vi "WriteLog.vi"(8 "Online Eye Model":T2, 10 "Current System State":T1(ring), 11 "File In":refnum<file>) -> (3 "File Out":refnum<file>)   [LabVIEW 2016]
uses:
  Subsystems/Global Variables.vi
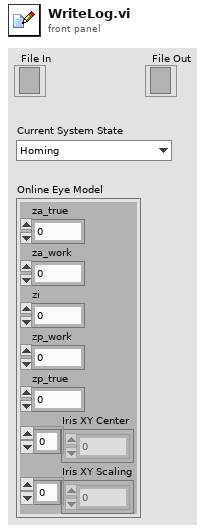
[diagram p1: front panel]
types:
  T1 = enum16{"Homing", "M/S Initialization", "M/S Operation", "Aiming", "Engaging", "Trajectory Loading", "Tracking Initialization", "Tracking", "Rerouting", "Regulation"}
  T2 = cluster{"za_true":dbl, "za_work":dbl, "zi":dbl, "zp_work":dbl, "zp_true":dbl, "Iris XY Center":dbl[], "Iris XY Scaling":dbl[]}
  T3 = cluster{"Accurus button":bool[], "Accurus engaged?":bool, "Vacuum Force":i32, "Accurus Ch. A Vout":dbl, "Accurus Ch. B Vout":dbl, "Irrigation engaged?":bool}
  T4 = cluster{"Iris XY Center[0]":dbl, "Iris XY Center[1]":dbl, "Iris XY Center[2]":dbl, "Iris XY Center[3]":dbl, "Iris XY Center[4]":dbl, "Iris XY Center[5]":dbl, "Iris XY Center[6]":dbl, "Iris XY Center[7]":dbl, "Iris XY Center[8]":dbl}
  T5 = cluster{"Iris XY Scaling[0]":dbl, "Iris XY Scaling[1]":dbl, "Iris XY Scaling[2]":dbl, "Iris XY Scaling[3]":dbl, "Iris XY Scaling[4]":dbl, "Iris XY Scaling[5]":dbl, "Iris XY Scaling[6]":dbl, "Iris XY Scaling[7]":dbl, "Iris XY Scaling[8]":dbl}
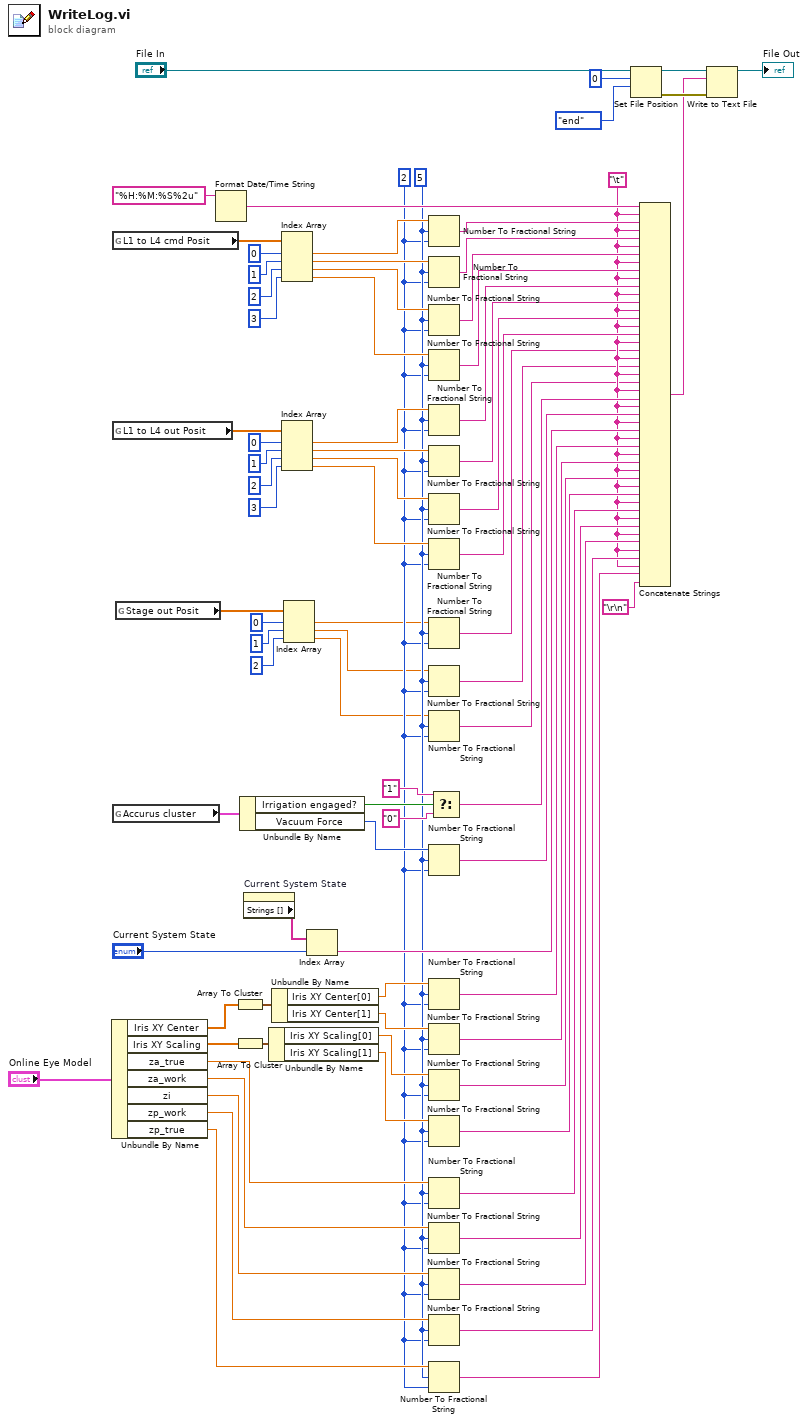
[diagram p0: block diagram]
diagram:
  w7 = 2
  w8 = 5
  w13 = "\t"
  n1 = Unbundle By Name("Online Eye Model") -> ("Iris XY Center"=w37:dbl[], "Iris XY Scaling"=w34:dbl[], "za_true"=w29:dbl, "za_work"=w28:dbl, "zi"=w27:dbl, "zp_work"=w26:dbl, "zp_true"=w25:dbl)
  n2 = global read "Global Variables.vi" "L1 to L4 cmd Posit"() -> (w69:dbl[])
  n3 = global read "Global Variables.vi" "L1 to L4 out Posit"() -> (w52:dbl[])
  n4 = global read "Global Variables.vi" "Accurus cluster"() -> (w47:T3)
  n5 = global read "Global Variables.vi" "Stage out Posit"() -> (w12:dbl[])
  n6 = Format Date/Time String(time format string (%c)="%H:%M:%S%2u") -> (date/time string=w74:string)  [unwired: 2 in]
  n7 = Array To Cluster(array=w37) -> (cluster=w36:T4)
  n8 = Array To Cluster(array=w34) -> (cluster=w35:T5)
  n9 = Unbundle By Name(w47) -> ("Irrigation engaged?"=w45:bool, "Vacuum Force"=w46:i32)
  n10 = property on="Current System State" class="Enum (strict)"() -> ("Strings []"=w41:string[])  [unwired: 2 in, 2 out]
  n11 = Unbundle By Name(w35) -> ("Iris XY Scaling[0]"=w31:dbl, "Iris XY Scaling[1]"=w30:dbl)
  n12 = Unbundle By Name(w36) -> ("Iris XY Center[0]"=w33:dbl, "Iris XY Center[1]"=w32:dbl)
  n13 = Index Array(array=w69, index #1=0 ("index"), index #2=1 ("index"), index #3=2 ("index"), index #4=3 ("index")) -> (element #1=w68:dbl, element #2=w61:dbl, element #3=w67:dbl, element #4=w66:dbl)
  n14 = Index Array(array=w52, index #1=0 ("index"), index #2=1 ("index"), index #3=2 ("index"), index #4=3 ("index")) -> (element #1=w54:dbl, element #2=w53:dbl, element #3=w59:dbl, element #4=w60:dbl)
  n15 = Index Array(array=w12, index #1=0 ("index"), index #2=1 ("index"), index #3=2 ("index")) -> (element #1=w6:dbl, element #2=w5:dbl, element #3=w4:dbl)
  n16 = Index Array(array=w41, index="Current System State") -> (element=w39:string)
  n17 = Number To Fractional String(number=w68, width (-)=w8, precision (6)=w7) -> (F-format string=w65:string)  [unwired: 1 in]
  n18 = Number To Fractional String(number=w61, width (-)=w8, precision (6)=w7) -> (F-format string=w64:string)  [unwired: 1 in]
  n19 = Number To Fractional String(number=w67, width (-)=w8, precision (6)=w7) -> (F-format string=w63:string)  [unwired: 1 in]
  n20 = Number To Fractional String(number=w66, width (-)=w8, precision (6)=w7) -> (F-format string=w62:string)  [unwired: 1 in]
  n21 = Number To Fractional String(number=w54, width (-)=w8, precision (6)=w7) -> (F-format string=w51:string)  [unwired: 1 in]
  n22 = Number To Fractional String(number=w53, width (-)=w8, precision (6)=w7) -> (F-format string=w50:string)  [unwired: 1 in]
  n23 = Number To Fractional String(number=w59, width (-)=w8, precision (6)=w7) -> (F-format string=w49:string)  [unwired: 1 in]
  n24 = Number To Fractional String(number=w60, width (-)=w8, precision (6)=w7) -> (F-format string=w48:string)  [unwired: 1 in]
  n25 = Number To Fractional String(number=w6, width (-)=w8, precision (6)=w7) -> (F-format string=w3:string)  [unwired: 1 in]
  n26 = Number To Fractional String(number=w5, width (-)=w8, precision (6)=w7) -> (F-format string=w2:string)  [unwired: 1 in]
  n27 = Number To Fractional String(number=w4, width (-)=w8, precision (6)=w7) -> (F-format string=w1:string)  [unwired: 1 in]
  n28 = Number To Fractional String(number=w46, width (-)=w8, precision (6)=w7) -> (F-format string=w42:string)  [unwired: 1 in]
  n29 = Number To Fractional String(number=w33, width (-)=w8, precision (6)=w7) -> (F-format string=w24:string)  [unwired: 1 in]
  n30 = Number To Fractional String(number=w32, width (-)=w8, precision (6)=w7) -> (F-format string=w23:string)  [unwired: 1 in]
  n31 = Number To Fractional String(number=w31, width (-)=w8, precision (6)=w7) -> (F-format string=w22:string)  [unwired: 1 in]
  n32 = Number To Fractional String(number=w30, width (-)=w8, precision (6)=w7) -> (F-format string=w21:string)  [unwired: 1 in]
  n33 = Number To Fractional String(number=w29, width (-)=w8, precision (6)=w7) -> (F-format string=w20:string)  [unwired: 1 in]
  n34 = Number To Fractional String(number=w28, width (-)=w8, precision (6)=w7) -> (F-format string=w19:string)  [unwired: 1 in]
  n35 = Number To Fractional String(number=w27, width (-)=w8, precision (6)=w7) -> (F-format string=w18:string)  [unwired: 1 in]
  n36 = Number To Fractional String(number=w26, width (-)=w8, precision (6)=w7) -> (F-format string=w17:string)  [unwired: 1 in]
  n37 = Number To Fractional String(number=w25, width (-)=w8, precision (6)=w7) -> (F-format string=w16:string)  [unwired: 1 in]
  n38 = Select(t="1" ("time format string (%c)"), s=w45, f="0" ("time format string (%c)")) -> (s? t:f=w14:string)
  n39 = Set File Position(offset (in bytes) (0)=i64 0, refnum="File In", from (0:start)=enum16{"start", "end", "current"}."end") -> (refnum out=w78:refnum<file>, error out=w77:errorcluster)  [unwired: 1 in]
  n40 = Concatenate Strings(w74, w13, w65, w13, w64, w13, w63, w13, w62, w13, w51, w13, w50, w13, w49, w13, w48, w13, w3, w13, w2, w13, w1, w13, w14, w13, w42, w13, w39, w13, w24, w13, w23, w13, w22, w13, w21, w13, w20, w13, w19, w13, w18, w13, w17, w13, w16, "\r\n") -> (w75:string)
  n41 = Write to Text File(file (use dialog)=w78, text=w75, error in=w77) -> (refnum out=→"File Out":refnum<file>)  [unwired: 1 in, 2 out]
